vi "decodeData.vi"(0 "Read Buffer":string) -> (1 "Acc X":sgl[](array[numeric]), 2 "AccY":sgl[](array[numeric]), 3 "AccZ":sgl[](array[numeric]), 4 "GyroX":sgl[](array[numeric]), 5 "Roll":sgl[](array[numeric]), 6 "GyroY":sgl[](array[numeric]), 7 "Pitch":sgl[](array[numeric]), 8 "GyroZ":sgl[](array[numeric]), 9 "Yaw":sgl[](array[numeric]), 10 "RwYc":sgl[](array[numeric]), 11 "RwXc":sgl[](array[numeric]), 12 "RwX":sgl[](array[numeric]), 13 "RwY":sgl[](array[numeric]), 14 "RwZ":sgl[](array[numeric]), 15 "RwZc":sgl[](array[numeric]))   [LabVIEW 2020]
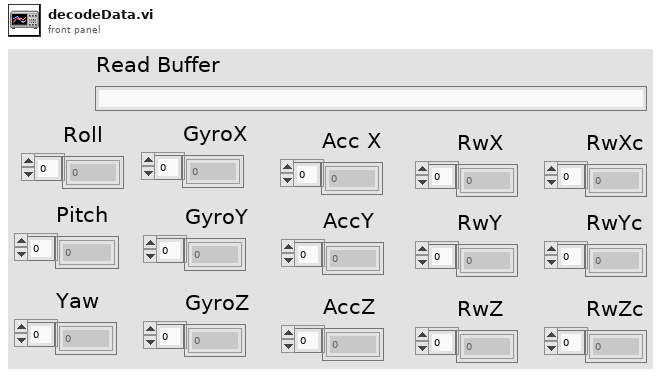
[diagram p1: front panel]
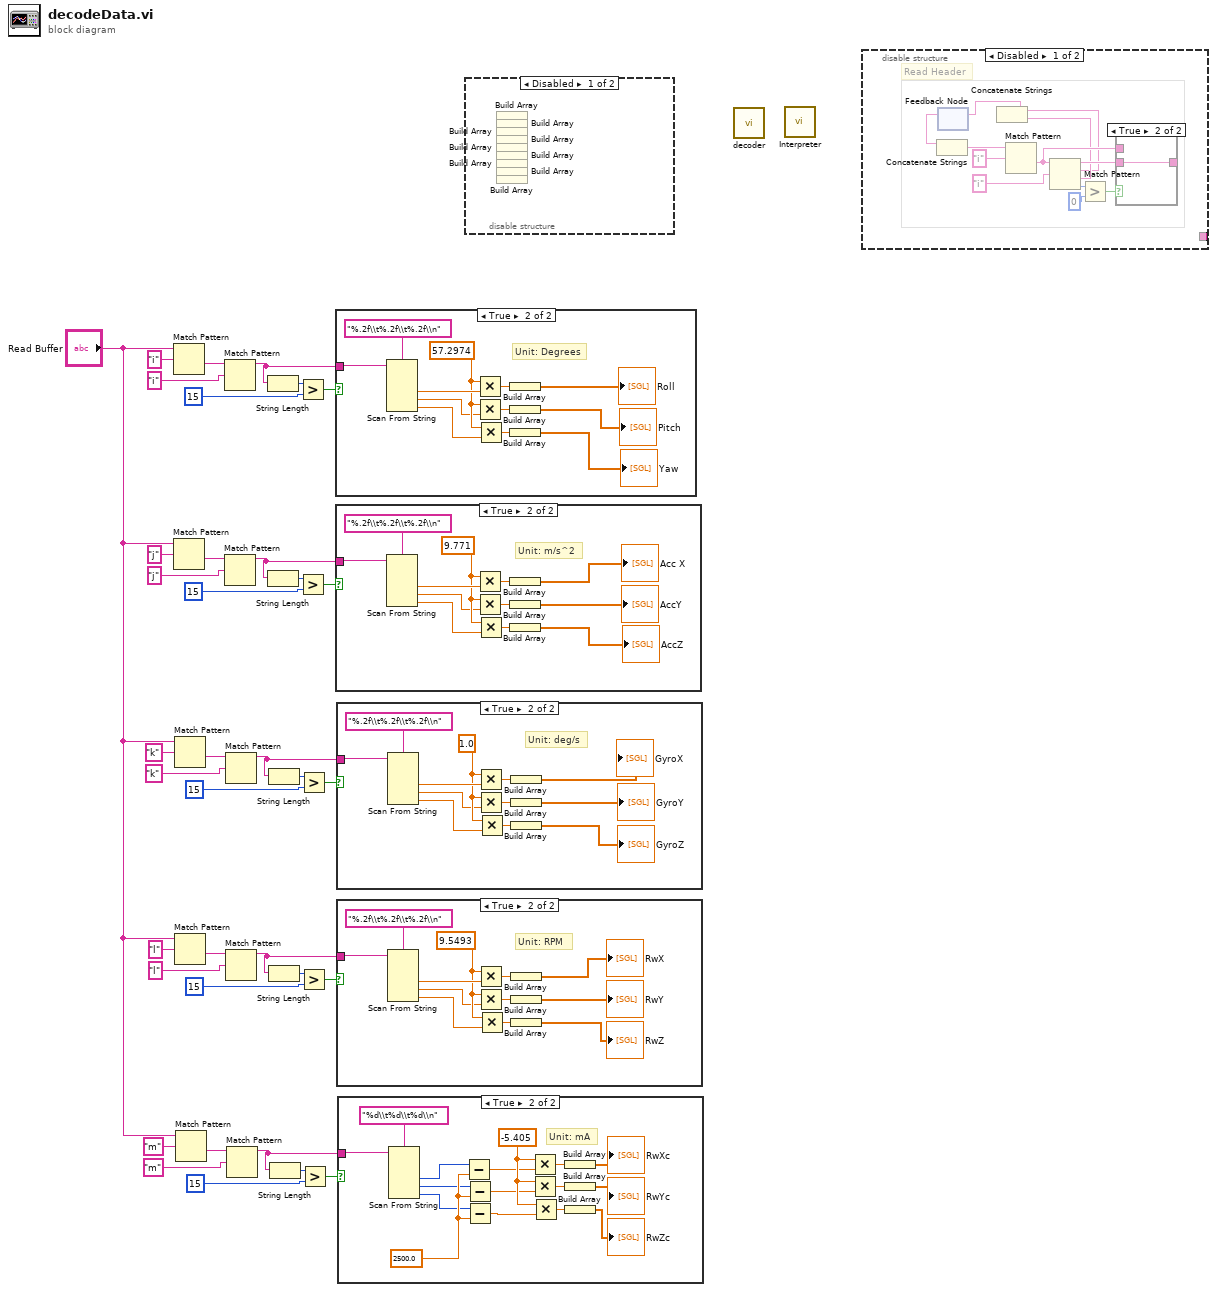
[diagram p0: block diagram]
diagram:
  n1 = Match Pattern(string="Read Buffer", regular expression="i") -> (after substring=w34:string)  [unwired: 1 in, 3 out]
  n2 = Match Pattern(string="Read Buffer", regular expression="j") -> (after substring=w27:string)  [unwired: 1 in, 3 out]
  n3 = Match Pattern(string="Read Buffer", regular expression="k") -> (after substring=w20:string)  [unwired: 1 in, 3 out]
  n4 = Match Pattern(string="Read Buffer", regular expression="l") -> (after substring=w13:string)  [unwired: 1 in, 3 out]
  n5 = Match Pattern(string="Read Buffer", regular expression="m") -> (after substring=w6:string)  [unwired: 1 in, 3 out]
  n6 = Match Pattern(string=w34, regular expression="i") -> (before substring=w33:string)  [unwired: 1 in, 3 out]
  n7 = Match Pattern(string=w27, regular expression="j") -> (before substring=w26:string)  [unwired: 1 in, 3 out]
  n8 = Match Pattern(string=w20, regular expression="k") -> (before substring=w19:string)  [unwired: 1 in, 3 out]
  n9 = Match Pattern(string=w13, regular expression="l") -> (before substring=w12:string)  [unwired: 1 in, 3 out]
  n10 = Match Pattern(string=w6, regular expression="m") -> (before substring=w5:string)  [unwired: 1 in, 3 out]
  n11 = String Length(string=w33) -> (length=w32:i32)
  n12 = String Length(string=w26) -> (length=w25:i32)
  n13 = String Length(string=w19) -> (length=w18:i32)
  n14 = String Length(string=w12) -> (length=w11:i32)
  n15 = String Length(string=w5) -> (length=w4:i32)
  n16 = Greater?(x=w32, y=15) -> (0:w30:bool)
  n17 = Greater?(x=w25, y=15) -> (0:w23:bool)
  n18 = Greater?(x=w18, y=15) -> (0:w16:bool)
  n19 = Greater?(x=w11, y=15) -> (0:w9:bool)
  n20 = Greater?(x=w4, y=15) -> (0:w2:bool)
  n21 = case shown="True" w30 {
    tunnel: w33 -> [_ w48]
    frame False {
    }
    frame True {
      w38 = 57.2974 ("x")
      # "Unit: Degrees"
      n22 = Scan From String(format string="%.2f\\t%.2f\\t%.2f\\n", input string=w48) -> (output 1=w43:dbl, output 2=w37:dbl, output 3=w40:dbl)  [unwired: 5 in, 3 out]
      n23 = Multiply(x=w38, y=w43) -> (x*y=w42:dbl)
      n24 = Multiply(x=w38, y=w37) -> (x*y=w39:dbl)
      n25 = Multiply(x=w38, y=w40) -> (x*y=w41:dbl)
      n26 = Build Array(w42) -> (→"Roll":dbl[])
      n27 = Build Array(w39) -> (→"Pitch":dbl[])
      n28 = Build Array(w41) -> (→"Yaw":dbl[])
    }
  }
  n29 = case shown="True" w23 {
    tunnel: w26 -> [_ w60]
    frame False {
    }
    frame True {
      w53 = 9.771 ("x")
      # "Unit: m/s^2"
      n30 = Scan From String(format string="%.2f\\t%.2f\\t%.2f\\n", input string=w60) -> (output 1=w58:dbl, output 2=w52:dbl, output 3=w55:dbl)  [unwired: 5 in, 3 out]
      n31 = Multiply(x=w53, y=w58) -> (x*y=w57:dbl)
      n32 = Multiply(x=w53, y=w52) -> (x*y=w54:dbl)
      n33 = Multiply(x=w53, y=w55) -> (x*y=w56:dbl)
      n34 = Build Array(w57) -> (→"Acc X":dbl[])
      n35 = Build Array(w54) -> (→"AccY":dbl[])
      n36 = Build Array(w56) -> (→"AccZ":dbl[])
    }
  }
  n37 = case shown="True" w16 {
    tunnel: w19 -> [_ w72]
    frame False {
    }
    frame True {
      w65 = 1.0 ("x")
      # "Unit: deg/s"
      n38 = Scan From String(format string="%.2f\\t%.2f\\t%.2f\\n", input string=w72) -> (output 1=w70:dbl, output 2=w64:dbl, output 3=w67:dbl)  [unwired: 5 in, 3 out]
      n39 = Multiply(x=w65, y=w70) -> (x*y=w69:dbl)
      n40 = Multiply(x=w65, y=w64) -> (x*y=w66:dbl)
      n41 = Multiply(x=w65, y=w67) -> (x*y=w68:dbl)
      n42 = Build Array(w69) -> (→"GyroX":dbl[])
      n43 = Build Array(w66) -> (→"GyroY":dbl[])
      n44 = Build Array(w68) -> (→"GyroZ":dbl[])
    }
  }
  n45 = case shown="True" w9 {
    tunnel: w12 -> [_ w84]
    frame False {
    }
    frame True {
      w77 = 9.5493 ("x")
      # "Unit: RPM"
      n46 = Scan From String(format string="%.2f\\t%.2f\\t%.2f\\n", input string=w84) -> (output 1=w82:dbl, output 2=w76:dbl, output 3=w79:dbl)  [unwired: 5 in, 3 out]
      n47 = Multiply(x=w77, y=w82) -> (x*y=w81:dbl)
      n48 = Multiply(x=w77, y=w76) -> (x*y=w78:dbl)
      n49 = Multiply(x=w77, y=w79) -> (x*y=w80:dbl)
      n50 = Build Array(w81) -> (→"RwX":dbl[])
      n51 = Build Array(w78) -> (→"RwY":dbl[])
      n52 = Build Array(w80) -> (→"RwZ":dbl[])
    }
  }
  n53 = case shown="True" w2 {
    tunnel: w5 -> [_ w100]
    frame False {
    }
    frame True {
      w91 = 2500.0 ("x")
      w95 = -5.405 ("x")
      # "Unit: mA"
      n54 = Scan From String(format string="%d\\t%d\\t%d\\n", input string=w100) -> (output 1=w90:i32, output 2=w89:i32, output 3=w88:i32)  [unwired: 5 in, 3 out]
      n55 = Subtract(x=w90, y=w91) -> (x-y=w87:dbl)
      n56 = Subtract(x=w89, y=w91) -> (x-y=w86:dbl)
      n57 = Subtract(x=w88, y=w91) -> (x-y=w85:dbl)
      n58 = Multiply(x=w95, y=w87) -> (x*y=w98:dbl)
      n59 = Multiply(x=w95, y=w86) -> (x*y=w96:dbl)
      n60 = Multiply(x=w95, y=w85) -> (x*y=w97:dbl)
      n61 = Build Array(w98) -> (→"RwXc":dbl[])
      n62 = Build Array(w96) -> (→"RwYc":dbl[])
      n63 = Build Array(w97) -> (→"RwZc":dbl[])
    }
  }
  n64 = disable-structure shown="Disabled" {
    frame Disabled {
      n65 = Build Array() -> ()  [unwired: 1 in, 1 out]
      n66 = Build Array() -> ()  [unwired: 1 in, 1 out]
      n67 = Build Array() -> ()  [unwired: 1 in, 1 out]
      n68 = Build Array() -> ()  [unwired: 1 in, 1 out]
      n69 = Build Array() -> ()  [unwired: 1 in, 1 out]
      n70 = Build Array() -> ()  [unwired: 1 in, 1 out]
      n71 = Build Array() -> ()  [unwired: 1 in, 1 out]
      n72 = Build Array() -> ()  [unwired: 1 in, 1 out]
      n73 = Build Array() -> ()  [unwired: 1 in, 1 out]
    }
    frame Enabled {
    }
  }
  n74 = call "decoder.vi"() -> ()  [unwired: 11 in, 1 out]
  n75 = call "Interpreter.vi"() -> ()  [unwired: 8 in, 12 out]
  n76 = disable-structure shown="Disabled" {
    disable-tunnel: _ -> [w114 _]
    frame Disabled {
      # "Read Header"
      n77 = feedback #1() -> (w109:string)  [unwired: 1 in]
      n78 = Concatenate Strings(w109) -> (w108:string, w113:string)
      n79 = Match Pattern(string=w108, regular expression="i") -> (after substring=w110:string)  [unwired: 1 in, 3 out]
      n80 = Match Pattern(string=w110, regular expression="i") -> (before substring=w111:string, match substring=w105:string, after substring=w106:string, offset past match=w107:i32)  [unwired: 1 in]
      n81 = Concatenate Strings(w105, w106) -> (w101:string)
      n82 = feedback-in #1(w101) -> ()
      n83 = Greater?(x=w107, y=0) -> (0:w112:bool)
      n84 = case shown="True" w112 {
        tunnel: [w115 w116] -> _
        tunnel: w111 -> [_ w116]
        tunnel: w110 -> [w115 _]
        frame False {
        }
        frame True {
        }
      }
    }
    frame Enabled {
    }
  }
